vi "Delete Script.vi"(8 "error in":errorcluster, 9 "Script Name":string, 11 "VISA resource name":refnum<visa-resource-name>) -> (0 "error out":errorcluster, 3 "VISA resource name out":refnum<visa-resource-name>, 4 "Command String":string)   [LabVIEW 2009, in "Keithley 2600 Series.lvlib"]
doc: "This VI deletes a user script from the instrument's non-volatile memory.\n\n<b>Functions and Attributes Used</b>\nscript.delete()"
uses:
  <instrlib>/Keithley 2600 Series/Keithley 2600 Series.lvlib
  <instrlib>/Keithley 2600 Series/Private/GlobalVariables.vi
panel:
  # "(c) 2008 Keithley Instruments, Inc.  ALL RIGHTS RESERVED."
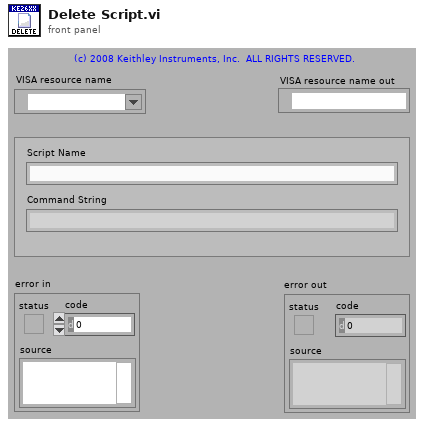
[diagram p1: front panel]
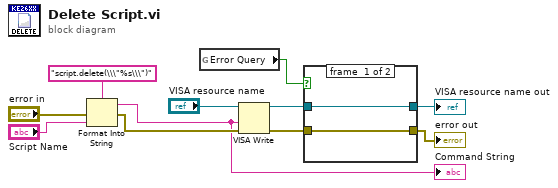
[diagram p0: block diagram]
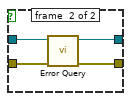
[diagram p2: hidden frame]
diagram:
  n1 = Format Into String(format string="script.delete(\\\"%s\\\")", error in="error in", "Script Name") -> (resulting string=w1:string, error out=w8:errorcluster)  [unwired: 1 in]
  "Command String" <- w1
  n2 = global read "GlobalVariables.vi" "Error Query"() -> (w6:bool)
  n3 = VISA Write(VISA resource name="VISA resource name", write buffer=w1, error in (no error)=w8) -> (VISA resource name out=w5:refnum<visa-resource-name>, error out=w4:errorcluster)  [unwired: 1 out]
  n4 = case shown="True" w6 {
    tunnel: w5 -> [w13 w17]
    tunnel: w4 -> [w12 w16]
    tunnel: [w13 w15] -> w3
    tunnel: [w12 w14] -> w2
    frame #0 {
    }
    frame #1 {
      n5 = call <instrlib>:"Error Query.vi"("error in (no error)"=w16, "VISA resource name"=w17) -> ("error out"=w14:errorcluster, "VISA resource name out"=w15:refnum<visa-resource-name>)  [unwired: 8 out]
    }
  }
  "VISA resource name out" <- w3
  "error out" <- w2
